vi "LM Three Gaussians and gradient.vi"(3 "output control":T1, 4 "data":variant, 5 "X":dbl[](array[numeric]), 6 "a":dbl[](array[numeric])) -> (0 "error out":errorcluster, 1 "f'(X,a)":dbl[][](array[numeric]), 2 "f(X,a)":dbl[](array[numeric]))   [LabVIEW 2019]
doc: "This template is the starting point for creating a model function to be passed to the Nonlinear Curve Fit.vi."
uses:
  <vilib>/gmath/NumericalOptimization/LM_output select.ctl
  ALiX/D-Only Fixed Parameters.ctl
  <vilib>/gmath/NI_Gmath.lvlib
panel:
  # "Parameters:\n\namplitude 1: A1\ncenter 1: t1\nSDV 1: s1\nAmplitude 2: A2\ncenter 2: t2\nSDV 2: s2\nAmplitude 3: A3\ncenter 3: t3\nSDV 3: s3"
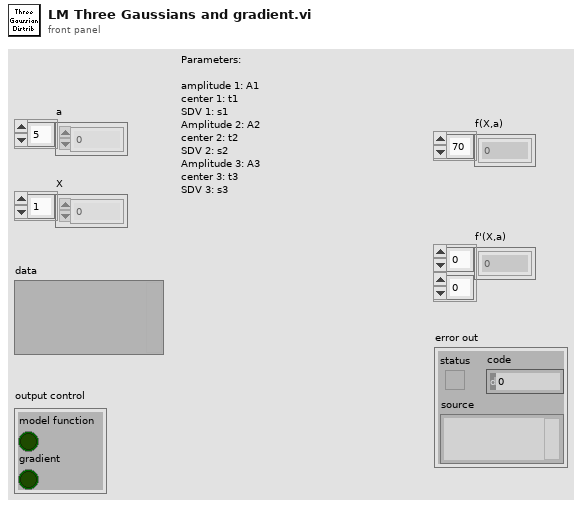
[diagram p1: front panel]
types:
  T1 = typedef "NI_Gmath.lvlib/LM_output select.ctl" = cluster{"model function":bool, "gradient":bool}
  T2 = typedef "D-Only Fixed Parameters.ctl" = cluster{"Fix D-only Peak Location":bool, "Peak Location":dbl, "Fix D-only Peak FWHM":bool, "Peak FWHM":dbl}
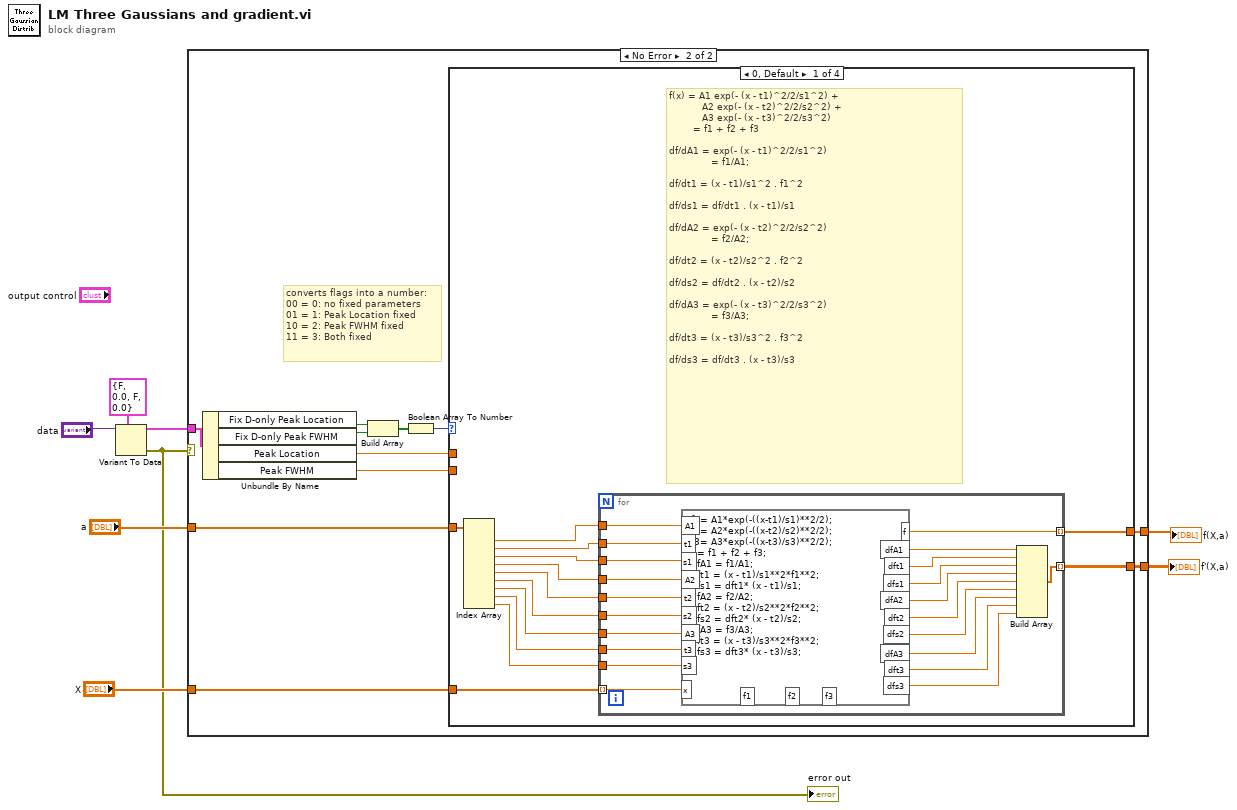
[diagram p0: block diagram]
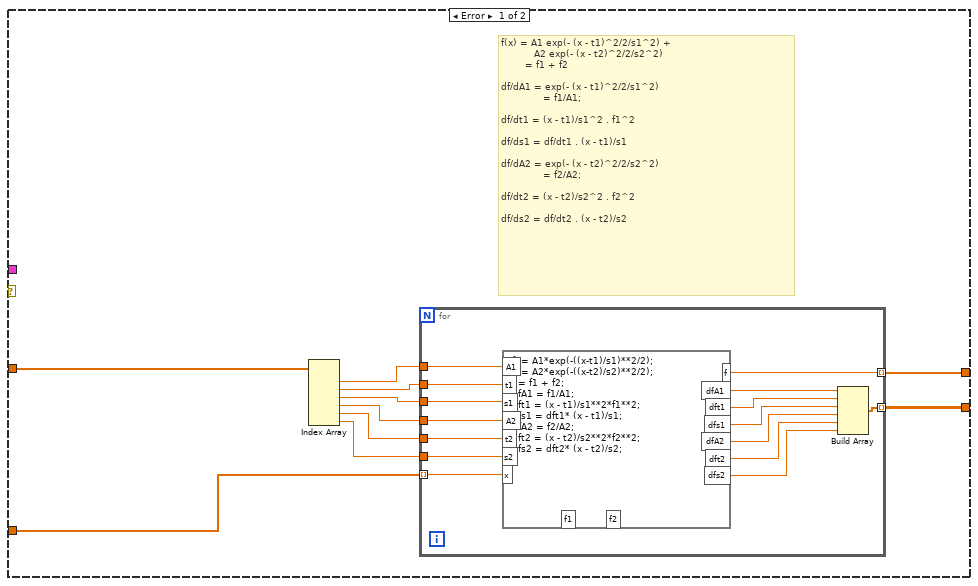
[diagram p2: hidden frame]
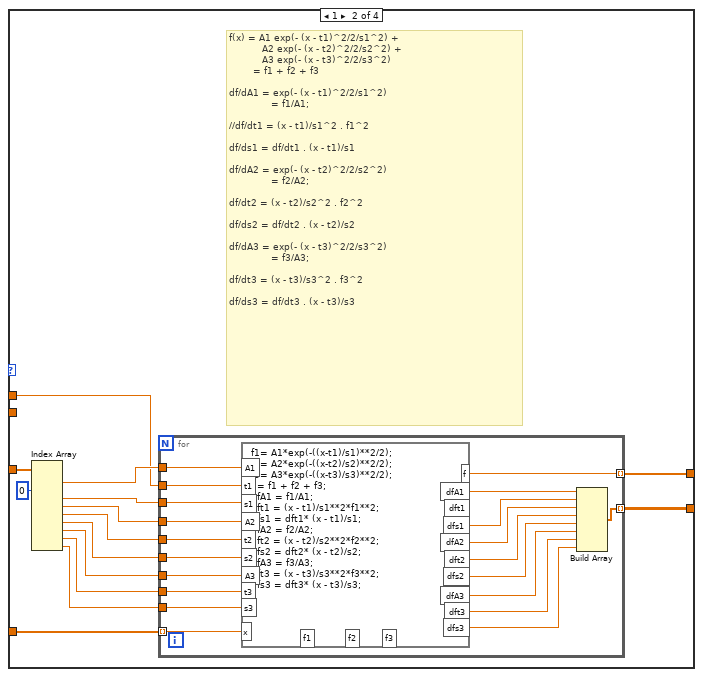
[diagram p3: hidden frame]
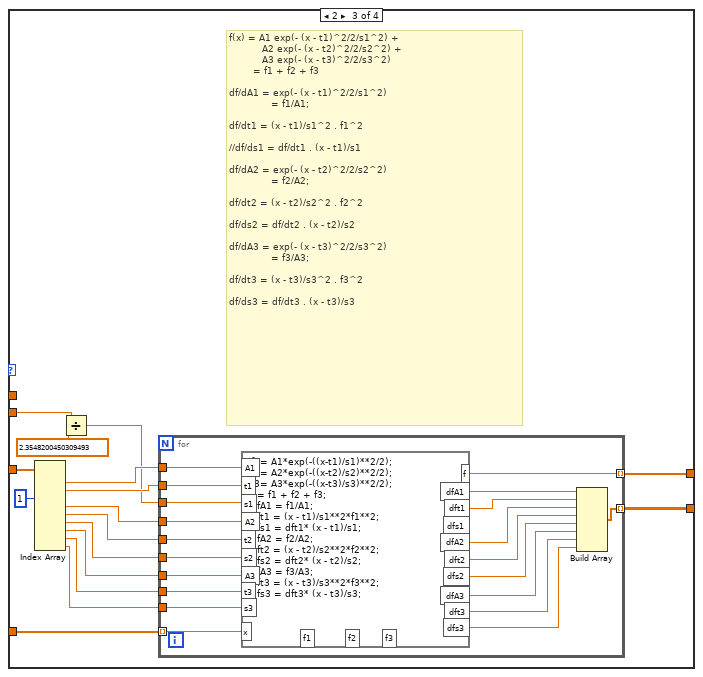
[diagram p4: hidden frame]
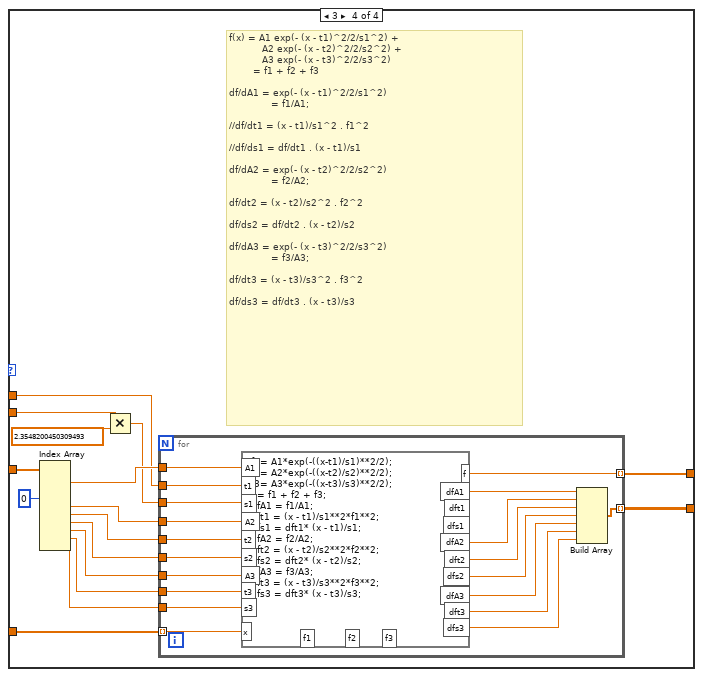
[diagram p5: hidden frame]
diagram:
  n1 = Variant To Data(type=T2 {"Fix D-only Peak Location"=FALSE, "Peak Location"=0.0, "Fix D-only Peak FWHM"=FALSE, "Peak FWHM"=0.0} ("Fixed Parameters"), Variant="data") -> (data=w2:T2, error out=w1:errorcluster)  [unwired: 1 in]
  "error out" <- w1
  n2 = case shown="No Error" w1 {
    tunnel: "a" -> [w18 w44]
    tunnel: "X" -> [w17 w43]
    tunnel: [w16 w42] -> w6
    tunnel: [w15 w41] -> w5
    tunnel: w2 -> [_ w40]
    frame Error {
      # "f(x) = A1 exp(- (x - t1)^2/2/s1^2) +\n           A2 exp(- (x - t2)^2/2/s2^2)\n        = f1 + f2\n\ndf/dA1 = exp(- (x - t1)^2/2/s1^2)\n              = f1/A1;\n\ndf/dt1 = (x - t1)/s1^2 . f1^2\n\ndf/ds1 = df/dt1 . (x - t1)/s1                     \n\ndf/dA2 = exp(- (x - t2)^2/2/s2^2)\n              = f2/A2;\n\ndf/dt2 = (x - t2)/s2^2 . f2^2\n\ndf/ds2 = df/dt2 . (x - t2)/s2"
      n3 = Index Array(array=w18) -> (element #1=w14:dbl, element #2=w13:dbl, element #3=w12:dbl, element #4=w11:dbl, element #5=w10:dbl, element #6=w9:dbl)  [unwired: 6 in]
      n4 = for {
        tunnel: w17 -> [w33] mode=indexing
        tunnel: [w31] -> w16 mode=indexing
        tunnel: [w30] -> w15 mode=indexing
        tunnel: w14 -> [w29]
        tunnel: w13 -> [w28]
        tunnel: w12 -> [w27]
        tunnel: w11 -> [w26]
        tunnel: w10 -> [w25]
        tunnel: w9 -> [w24]
        n5 = formula code="f1= A1*exp(-((x-t1)/s1)**2/2);\nf2= A2*exp(-((x-t2)/s2)**2/2);\nf = f1 + f2;\ndfA1 = f1/A1;\ndft1 = (x - t1)/s1**2*f1**2;\ndfs1 = dft1* (x - t1)/s1;\ndfA2 = f2/A2;\ndft2 = (x - t2)/s2**2*f2**2;\ndfs2 = dft2* (x - t2)/s2;"("A1"=w29, "t1"=w28, "s1"=w27, "x"=w33, "A2"=w26, "t2"=w25, "s2"=w24) -> ("f"=w31:dbl, "dfA1"=w32:dbl, "dft1"=w23:dbl, "dfs1"=w22:dbl, "dfA2"=w21:dbl, "dft2"=w20:dbl, "dfs2"=w19:dbl)  [unwired: 2 out]
        n6 = Build Array(w32, w23, w22, w21, w20, w19) -> (w30:dbl[])
      }
    }
    frame No Error {
      # "converts flags into a number:\n00 = 0: no fixed parameters\n01 = 1: Peak Location fixed\n10 = 2: Peak FWHM fixed\n11 = 3: Both fixed"
      n7 = Unbundle By Name(w40) -> ("Fix D-only Peak Location"=w39:bool, "Fix D-only Peak FWHM"=w38:bool, "Peak Location"=w35:dbl, "Peak FWHM"=w34:dbl)
      n8 = Build Array(w39, w38) -> (w37:bool[])
      n9 = Boolean Array To Number(Boolean array=w37) -> (number=w36:u32)
      n10 = case shown="0, Default" w36 {
        tunnel: w44 -> [w57 w92 w128 w164]
        tunnel: w43 -> [w56 w91 w127 w163]
        tunnel: [w55 w90 w126 w162] -> w42
        tunnel: [w54 w89 w125 w161] -> w41
        tunnel: w35 -> [_ w79 _ w153]
        tunnel: w34 -> [_ _ w114 w152]
        frame 0, Default {
          # "f(x) = A1 exp(- (x - t1)^2/2/s1^2) +\n           A2 exp(- (x - t2)^2/2/s2^2) +\n           A3 exp(- (x - t3)^2/2/s3^2)\n        = f1 + f2 + f3\n\ndf/dA1 = exp(- (x - t1)^2/2/s1^2)\n              = f1/A1;\n\ndf/dt1 = (x - t1)/s1^2 . f1^2\n\ndf/ds1 = df/dt1 . (x - t1)/s1                     \n\ndf/dA2 = exp(- (x - t2)^2/2/s2^2)\n              = f2/A2;\n\ndf/dt2 = (x - t2)/s2^2 . f2^2\n\ndf/ds2 = df/dt2 . (x - t2)/s2                     \n\ndf/dA3 = exp(- (x - t3)^2/2/s3^2)\n              = f3/A3;\n\ndf/dt3 = (x - t3)/s3^2 . f3^2\n\ndf/ds3 = df/dt3 . (x - t3)/s3"
          n11 = Index Array(array=w57) -> (element #1=w53:dbl, element #2=w52:dbl, element #3=w51:dbl, element #4=w50:dbl, element #5=w49:dbl, element #6=w48:dbl, element #7=w47:dbl, element #8=w46:dbl, element #9=w45:dbl)  [unwired: 9 in]
          n12 = for {
            tunnel: w56 -> [w78] mode=indexing
            tunnel: [w76] -> w55 mode=indexing
            tunnel: [w75] -> w54 mode=indexing
            tunnel: w53 -> [w74]
            tunnel: w52 -> [w73]
            tunnel: w51 -> [w72]
            tunnel: w50 -> [w71]
            tunnel: w49 -> [w70]
            tunnel: w48 -> [w69]
            tunnel: w47 -> [w63]
            tunnel: w46 -> [w62]
            tunnel: w45 -> [w61]
            n13 = formula code="f1= A1*exp(-((x-t1)/s1)**2/2);\nf2= A2*exp(-((x-t2)/s2)**2/2);\nf3= A3*exp(-((x-t3)/s3)**2/2);\nf = f1 + f2 + f3;\ndfA1 = f1/A1;\ndft1 = (x - t1)/s1**2*f1**2;\ndfs1 = dft1* (x - t1)/s1;\ndfA2 = f2/A2;\ndft2 = (x - t2)/s2**2*f2**2;\ndfs2 = dft2* (x - t2)/s2; \ndfA3 = f3/A3;\ndft3 = (x - t3)/s3**2*f3**2;\ndfs3 = dft3* (x - t3)/s3;"("A1"=w74, "t1"=w73, "s1"=w72, "x"=w78, "A2"=w71, "t2"=w70, "s2"=w69, "A3"=w63, "t3"=w62, "s3"=w61) -> ("f"=w76:dbl, "dfA1"=w77:dbl, "dft1"=w68:dbl, "dfs1"=w67:dbl, "dfA2"=w66:dbl, "dft2"=w65:dbl, "dfs2"=w64:dbl, "dfA3"=w60:dbl, "dft3"=w59:dbl, "dfs3"=w58:dbl)  [unwired: 3 out]
            n14 = Build Array(w77, w68, w67, w66, w65, w64, w60, w59, w58) -> (w75:dbl[])
          }
        }
        frame 1 {
          # "f(x) = A1 exp(- (x - t1)^2/2/s1^2) +\n           A2 exp(- (x - t2)^2/2/s2^2) +\n           A3 exp(- (x - t3)^2/2/s3^2)\n        = f1 + f2 + f3\n\ndf/dA1 = exp(- (x - t1)^2/2/s1^2)\n              = f1/A1;\n\n//df/dt1 = (x - t1)/s1^2 . f1^2\n\ndf/ds1 = df/dt1 . (x - t1)/s1                     \n\ndf/dA2 = exp(- (x - t2)^2/2/s2^2)\n              = f2/A2;\n\ndf/dt2 = (x - t2)/s2^2 . f2^2\n\ndf/ds2 = df/dt2 . (x - t2)/s2                     \n\ndf/dA3 = exp(- (x - t3)^2/2/s3^2)\n              = f3/A3;\n\ndf/dt3 = (x - t3)/s3^2 . f3^2\n\ndf/ds3 = df/dt3 . (x - t3)/s3"
          n15 = Index Array(array=w92, index #2=0 ("index")) -> (element #1=w88:dbl, element #3=w87:dbl, element #4=w86:dbl, element #5=w85:dbl, element #6=w84:dbl, element #7=w83:dbl, element #8=w82:dbl, element #9=w81:dbl)  [unwired: 8 in, 1 out]
          n16 = for {
            tunnel: w91 -> [w112] mode=indexing
            tunnel: [w110] -> w90 mode=indexing
            tunnel: [w109] -> w89 mode=indexing
            tunnel: w88 -> [w108]
            tunnel: w79 -> [w107]
            tunnel: w87 -> [w106]
            tunnel: w86 -> [w105]
            tunnel: w85 -> [w104]
            tunnel: w84 -> [w103]
            tunnel: w83 -> [w98]
            tunnel: w82 -> [w97]
            tunnel: w81 -> [w96]
            n17 = formula code="f1= A1*exp(-((x-t1)/s1)**2/2);\nf2= A2*exp(-((x-t2)/s2)**2/2);\nf3= A3*exp(-((x-t3)/s3)**2/2);\nf = f1 + f2 + f3;\ndfA1 = f1/A1;\ndft1 = (x - t1)/s1**2*f1**2;\ndfs1 = dft1* (x - t1)/s1;\ndfA2 = f2/A2;\ndft2 = (x - t2)/s2**2*f2**2;\ndfs2 = dft2* (x - t2)/s2; \ndfA3 = f3/A3;\ndft3 = (x - t3)/s3**2*f3**2;\ndfs3 = dft3* (x - t3)/s3;"("A1"=w108, "t1"=w107, "s1"=w106, "x"=w112, "A2"=w105, "t2"=w104, "s2"=w103, "A3"=w98, "t3"=w97, "s3"=w96) -> ("f"=w110:dbl, "dfA1"=w111:dbl, "dfs1"=w102:dbl, "dfA2"=w101:dbl, "dft2"=w100:dbl, "dfs2"=w99:dbl, "dfA3"=w95:dbl, "dft3"=w94:dbl, "dfs3"=w93:dbl)  [unwired: 4 out]
            n18 = Build Array(w111, w102, w101, w100, w99, w95, w94, w93) -> (w109:dbl[])
          }
        }
        frame 2 {
          # "f(x) = A1 exp(- (x - t1)^2/2/s1^2) +\n           A2 exp(- (x - t2)^2/2/s2^2) +\n           A3 exp(- (x - t3)^2/2/s3^2)\n        = f1 + f2 + f3\n\ndf/dA1 = exp(- (x - t1)^2/2/s1^2)\n              = f1/A1;\n\ndf/dt1 = (x - t1)/s1^2 . f1^2\n\n//df/ds1 = df/dt1 . (x - t1)/s1                     \n\ndf/dA2 = exp(- (x - t2)^2/2/s2^2)\n              = f2/A2;\n\ndf/dt2 = (x - t2)/s2^2 . f2^2\n\ndf/ds2 = df/dt2 . (x - t2)/s2                     \n\ndf/dA3 = exp(- (x - t3)^2/2/s3^2)\n              = f3/A3;\n\ndf/dt3 = (x - t3)/s3^2 . f3^2\n\ndf/ds3 = df/dt3 . (x - t3)/s3"
          n19 = Index Array(array=w128, index #3=1 ("index")) -> (element #1=w124:dbl, element #2=w123:dbl, element #4=w122:dbl, element #5=w121:dbl, element #6=w120:dbl, element #7=w119:dbl, element #8=w118:dbl, element #9=w117:dbl)  [unwired: 8 in, 1 out]
          n20 = Divide(x=w114, y=2.3548200450309493) -> (x/y=w113:dbl)
          n21 = for {
            tunnel: w127 -> [w148] mode=indexing
            tunnel: [w146] -> w126 mode=indexing
            tunnel: [w145] -> w125 mode=indexing
            tunnel: w124 -> [w144]
            tunnel: w123 -> [w143]
            tunnel: w113 -> [w142]
            tunnel: w122 -> [w141]
            tunnel: w121 -> [w140]
            tunnel: w120 -> [w139]
            tunnel: w119 -> [w134]
            tunnel: w118 -> [w133]
            tunnel: w117 -> [w132]
            n22 = formula code="f1= A1*exp(-((x-t1)/s1)**2/2);\nf2= A2*exp(-((x-t2)/s2)**2/2);\nf3= A3*exp(-((x-t3)/s3)**2/2);\nf = f1 + f2 + f3;\ndfA1 = f1/A1;\ndft1 = (x - t1)/s1**2*f1**2;\ndfs1 = dft1* (x - t1)/s1;\ndfA2 = f2/A2;\ndft2 = (x - t2)/s2**2*f2**2;\ndfs2 = dft2* (x - t2)/s2; \ndfA3 = f3/A3;\ndft3 = (x - t3)/s3**2*f3**2;\ndfs3 = dft3* (x - t3)/s3;"("A1"=w144, "t1"=w143, "s1"=w142, "x"=w148, "A2"=w141, "t2"=w140, "s2"=w139, "A3"=w134, "t3"=w133, "s3"=w132) -> ("f"=w146:dbl, "dfA1"=w147:dbl, "dft1"=w138:dbl, "dfA2"=w137:dbl, "dft2"=w136:dbl, "dfs2"=w135:dbl, "dfA3"=w131:dbl, "dft3"=w130:dbl, "dfs3"=w129:dbl)  [unwired: 4 out]
            n23 = Build Array(w147, w138, w137, w136, w135, w131, w130, w129) -> (w145:dbl[])
          }
        }
        frame 3 {
          # "f(x) = A1 exp(- (x - t1)^2/2/s1^2) +\n           A2 exp(- (x - t2)^2/2/s2^2) +\n           A3 exp(- (x - t3)^2/2/s3^2)\n        = f1 + f2 + f3\n\ndf/dA1 = exp(- (x - t1)^2/2/s1^2)\n              = f1/A1;\n\n//df/dt1 = (x - t1)/s1^2 . f1^2\n\n//df/ds1 = df/dt1 . (x - t1)/s1                     \n\ndf/dA2 = exp(- (x - t2)^2/2/s2^2)\n              = f2/A2;\n\ndf/dt2 = (x - t2)/s2^2 . f2^2\n\ndf/ds2 = df/dt2 . (x - t2)/s2                     \n\ndf/dA3 = exp(- (x - t3)^2/2/s3^2)\n              = f3/A3;\n\ndf/dt3 = (x - t3)/s3^2 . f3^2\n\ndf/ds3 = df/dt3 . (x - t3)/s3"
          n24 = Index Array(array=w164, index #3=0 ("index")) -> (element #1=w160:dbl, element #4=w159:dbl, element #5=w158:dbl, element #6=w157:dbl, element #7=w156:dbl, element #8=w155:dbl, element #9=w154:dbl)  [unwired: 8 in, 2 out]
          n25 = Multiply(x=w152, y=2.3548200450309493) -> (x*y=w150:dbl)
          n26 = for {
            tunnel: w163 -> [w183] mode=indexing
            tunnel: [w181] -> w162 mode=indexing
            tunnel: [w180] -> w161 mode=indexing
            tunnel: w160 -> [w179]
            tunnel: w153 -> [w178]
            tunnel: w150 -> [w177]
            tunnel: w159 -> [w176]
            tunnel: w158 -> [w175]
            tunnel: w157 -> [w174]
            tunnel: w156 -> [w170]
            tunnel: w155 -> [w169]
            tunnel: w154 -> [w168]
            n27 = formula code="f1= A1*exp(-((x-t1)/s1)**2/2);\nf2= A2*exp(-((x-t2)/s2)**2/2);\nf3= A3*exp(-((x-t3)/s3)**2/2);\nf = f1 + f2 + f3;\ndfA1 = f1/A1;\ndft1 = (x - t1)/s1**2*f1**2;\ndfs1 = dft1* (x - t1)/s1;\ndfA2 = f2/A2;\ndft2 = (x - t2)/s2**2*f2**2;\ndfs2 = dft2* (x - t2)/s2; \ndfA3 = f3/A3;\ndft3 = (x - t3)/s3**2*f3**2;\ndfs3 = dft3* (x - t3)/s3;"("A1"=w179, "t1"=w178, "s1"=w177, "x"=w183, "A2"=w176, "t2"=w175, "s2"=w174, "A3"=w170, "t3"=w169, "s3"=w168) -> ("f"=w181:dbl, "dfA1"=w182:dbl, "dfA2"=w173:dbl, "dft2"=w172:dbl, "dfs2"=w171:dbl, "dfA3"=w167:dbl, "dft3"=w166:dbl, "dfs3"=w165:dbl)  [unwired: 5 out]
            n28 = Build Array(w182, w173, w172, w171, w167, w166, w165) -> (w180:dbl[])
          }
        }
      }
    }
  }
  "f(X,a)" <- w6
  "f'(X,a)" <- w5
